vi "HandleMenu.vi"(7 "Main Queue":T1, 8 "error in":errorcluster, 9 "Item Path":string, 10 "ItemTag":string, 11 "CEF_Repository in":refnum<class "CEF_Repository.lvclass">) -> (0 "error out":errorcluster, 2 "handled?":bool, 3 "CEF_Repository out":refnum<class "CEF_Repository.lvclass">)   [LabVIEW 2023, in "CEF.lvlib" / "CEF_Repository.lvclass"]
doc: "Copyright 2017 National Instruments Corporation\n\nLicensed under the Apache License, Version 2.0 (the \"License\"); you may not use this file except in compliance with the License. You may obtain a copy of the License at http://www.apache.org/licenses/LICENSE-2.0\nUnless required by applicable law or agreed to in writing, software distributed under the License is distributed on an \"AS IS\" BASIS, WITHOUT WARRANTIES OR CONDITIONS OF ANY KIND, either express or implied. See the License for the specific language governing permissions and limitations under the License."
uses:
  CEF_Repository.lvclass
  Node/mainQref.ctl
  Node/CEF_Node.lvclass
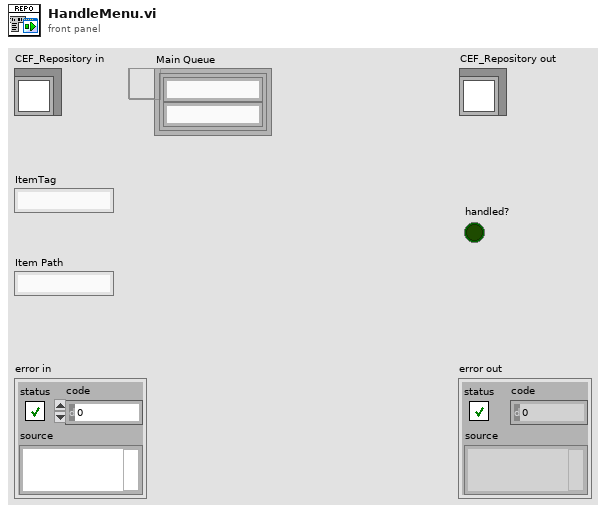
[diagram p1: front panel]
types:
  T1 = typedef "CEF.lvlib/CEF_Node.lvclass/mainQref.ctl" = refnum<queue>
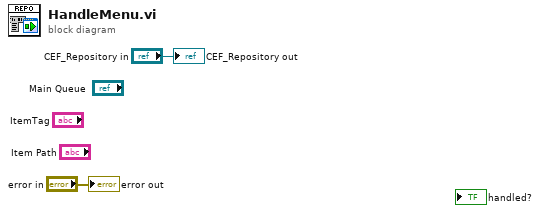
[diagram p0: block diagram]
diagram:
  "error out" <- "error in"
  "CEF_Repository out" <- "CEF_Repository in"
